vi "Close File Descriptor.vi"(8 "error in (no error)":errorcluster, 11 "Shared Memory in":refnum<class "Shared Memory.lvclass">) -> (0 "error out":errorcluster, 3 "Shared Memory out":refnum<class "Shared Memory.lvclass">)   [LabVIEW 2013, in "Linux RT IPC.Shared Memory.lvlib" / "Shared Memory.lvclass"]
doc: "This VI checks if a file descriptor is currently open. If so, it attemps to close the file descriptor using close()."
uses:
  Shared Memory.lvclass
  Shared Memory.lvclass/Shared Memory.ctl
  C/SubVIs/error handler.vi
  <vilib>/NI/NI Linux RT Errno/VIs/Public/Get Errno Value for Calling Thread.vi
  C/Linux RT IPC.C.lvlib
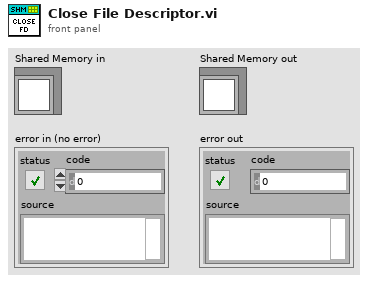
[diagram p1: front panel]
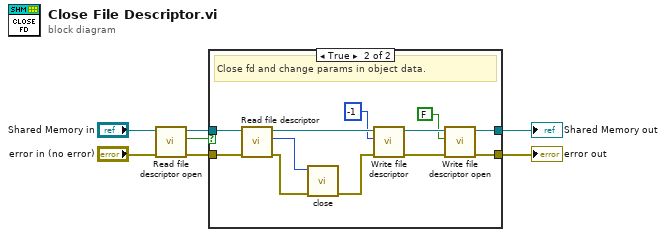
[diagram p0: block diagram]
diagram:
  n1 = call "Read file descriptor open.vi"("error in (no error)"="error in (no error)", "Shared Memory in"="Shared Memory in") -> ("error out"=w3:errorcluster, "file descriptor open"=w2:bool, "Shared Memory out"=w1:refnum<class "Shared Memory.lvclass">)  [unwired: 7 in]
  n2 = case shown="True" w2 {
    tunnel: w1 -> [w9 w21]
    tunnel: [w9 w11] -> w6
    tunnel: w3 -> [w8 w20]
    tunnel: [w8 w10] -> w7
    frame False {
      # "File descriptor is not open. Do nothing."
    }
    frame True {
      # "Close fd and change params in object data."
      n3 = call "Read file descriptor.vi"("error in (no error)"=w20, "Shared Memory in"=w21) -> ("error out"=w19:errorcluster, "file descriptor"=w18:i32, "Shared Memory out"=w17:refnum<class "Shared Memory.lvclass">)  [unwired: 7 in]
      n4 = call "close.vi"("error in (no error)"=w19, "file descriptor in"=w18) -> ("error out"=w16:errorcluster)  [unwired: 9 in]
      n5 = call "Write file descriptor.vi"("error in (no error)"=w16, "file descriptor"=-1, "Shared Memory in"=w17) -> ("error out"=w13:errorcluster, "Shared Memory out"=w14:refnum<class "Shared Memory.lvclass">)  [unwired: 7 in]
      n6 = call "Write file descriptor open.vi"("error in (no error)"=w13, "file descriptor open"=FALSE, "Shared Memory in"=w14) -> ("error out"=w10:errorcluster, "Shared Memory out"=w11:refnum<class "Shared Memory.lvclass">)  [unwired: 7 in]
    }
  }
  "error out" <- w7
  "Shared Memory out" <- w6
